vi "Turnaround.vi"(8 "error in (no error)":errorcluster) -> (0 "error out":errorcluster)   [LabVIEW 2016]
uses:
  Controls/Command cluster.ctl
  Controls/Command list.ctl
  Controls/Actuator fgv modes.ctl
  General/Controls/State control cluster.ctl
  General/Controls/States.ctl
  General/Controls/Queue modes.ctl
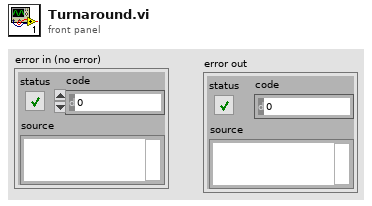
[diagram p1: front panel]
types:
  T1 = typedef "Queue modes.ctl" = enum16{"Initialise", "Destroy", "Get"}
  T2 = typedef "State control cluster.ctl" = cluster{"State":T3, "Data":variant}
  T3 = typedef "States.ctl" = enum16{"Initialise", "Actuator connection", "Get info", "Send command", "Load method", "Run method", "Save test", "Setup", "Shutdown"}
  T4 = typedef "Actuator fgv modes.ctl" = enum16{"Initalise", "COM", "Limit", "Speed", "Home", "Get"}
  T5 = typedef "Command cluster.ctl" = cluster{"Command":T6, "data":variant}
  T6 = typedef "Command list.ctl" = enum16{"", "£nabort", "getaxisno", "£getserialno", "£nidentify", "&&£setnlimit", "&£nm", "&£snv", "&£speed", "£np", "£ncal"}
  T7 = typedef "Default settings.ctl" = cluster{"COM port":refnum<visa-resource-name>, "Home pos":dbl, "Speed":dbl, "Limit stop":dbl}
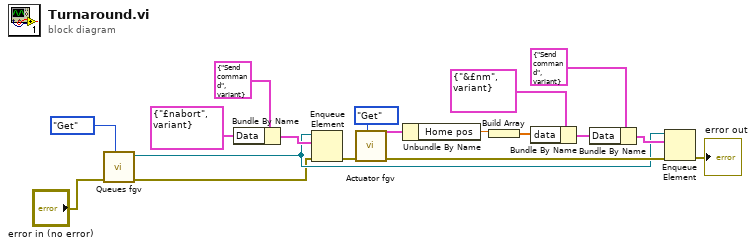
[diagram p0: block diagram]
diagram:
  n1 = call "Queues fgv.vi"("Modes"=Queue_modes."Get", "error in (no error)"="error in (no error)") -> ("error in (no error) 2"=w1:errorcluster, "Ivium"=w3:refnum<queue>)  [unwired: 6 in, 2 out]
  n2 = Bundle By Name(cluster=T2 {"State"=enum."Send command", "Data"=variant} ("element"), "Data"=T5 {"Command"=enum."£nabort", "data"=variant} ("Cluster")) -> (w11:T2)
  n3 = Enqueue Element(queue=w3, element=w11, error in (no error)=w1) -> (error out=w12:errorcluster)  [unwired: 1 in, 2 out]
  n4 = call "Actuator fgv.vi"("Enum"=Actuator_fgv_modes."Get", "error in (no error)"=w12) -> ("error out"=w17:errorcluster, "Cluster out"=w9:T7)  [unwired: 8 in]
  n5 = Unbundle By Name(w9) -> ("Home pos"=w10:dbl)
  n6 = Build Array(w10) -> (w14:dbl[])
  n7 = Bundle By Name(cluster=T5 {"Command"=enum."&£nm", "data"=variant} ("Cluster"), "data"=w14) -> (w16:T5)
  n8 = Bundle By Name(cluster=T2 {"State"=enum."Send command", "Data"=variant} ("element"), "Data"=w16) -> (w18:T2)
  n9 = Enqueue Element(queue=w3, element=w18, error in (no error)=w17) -> (error out=→"error out":errorcluster)  [unwired: 1 in, 2 out]
